vi "SwitchToAnalogOrDigital.vi"(0 "System no.":i32=1 min=1 step=1, 1 "Controller analog board":enum16{"E-711.iA4"}(ring), 2 "Axes to command":string[](array[string]), 3 "Mode":bool=TRUE caption="Mode (Analog:T)", 5 "error in":errorcluster, 6 "AI channels":dbl[](array[numeric]), 7 "AO channels":dbl[](array[numeric]), 8 "Lower voltage limit (V)":dbl=-10.0 format="%.6f", 9 "Upper voltage limit (V)":dbl=10.0 format="%.6f") -> (14 "Conversion factor":dbl[](array[numeric]) format="%.2f", 15 "Offset":dbl[](array[numeric]) format="%#.6f", 19 "Error out":errorcluster)   [LabVIEW 2014, in "PiFOC.lvlib"]
doc: "This VI sets communication parameters for analog or digital control. Run XXXX_Configuration_Setup.vi (with XXXX being the product number of your PI controller) prior to running this VI. \n\n¢ Set System no. to the same value as selected in XXXX_Configuration_ Setup.vi. \n¢ Select the name of the controller analog board (E-711.iA4).\n¢ Mode can be Analog (T) or Digital (F). \n¢ Lower voltage limit (V) and Upper voltage limit (V) must match the corresponding settings in Analog_Configuration_Setup.vi, representing the voltage range of the analog input of the controller. The VI checks if the selected values fit into the analog input voltage range of the controller. \n¢ Axes to command must be a sub set of the axes connected to the controller. \n¢ AI channels are the analog input channels of the controller to use for analog control. In contrast to the firmware internal names of the analog input channels, select \"1\" here for the first analog input, \"2\" for the second and so on. The VI will automatically determine which input channel names correspond to the selected analog input channels. \n¢ Similarly, select \"1\" for the first analog output channel (AO channels), \"2\" for the second analog output channel and so on, as the VI will automatically determine which output channel names correspond to the selected analog output channels. \n\nIf the current command level is 0 (CCL?), the VI switches to command level 1 (CCL) before making any further settings and back to 0 afterwards. \nWhen Analog is selected as Mode, the VI connects the selected analog input channels to the selected axes (SPA), sets gain and offset for the analog input (SPA), sets the output type to sensor monitor output (SPA), connects the selected analog output channels to the selected axes (SPA), and sets the position report scaling value and offset for the analog output (SPA).\nWhen Digital is selected as Mode, the VI disconnects the selected analog input channels from the axes (SPA) and sets the output type to control output (SPA).\nThe VI returns the total number of input and output channels available for this controller, the number of sensor input/output channels and the resulting number of analog input/output channels available for analog control. Also, it returns the Gain, Offset and Conversion factor settings resulting from the motion range (TMX?, TMN?) of the selected axes and sets the corresponding parameters (SPA). Finally, it returns the minimum and maximum analog input voltages of the controller as the given lower and upper voltage limits must fit into this range.\n\nSee XXXX_Sample_Application_With_Analog.vi (with XXXX being the product number of your PI controller) as a sample VI showing how to use this VI in combination with the corresponding Configuration_Setup VIs. \n\nValid for: E-709, E-712, E-725\n\nE-709: Controller analog board selection is E-711.iA4 (but board has different product code). \nE-712: Controller analog board is E-711.iA\nE-725: Controller analog board selection is E-711.iA4 (but board has different product code)."
uses:
  PiFOC.lvlib
panel:
  out "Max. controller\nanalog input voltage":dbl format="%#.6f"
  out "Min. controller\nanalog input voltage":dbl format="%#.6f"
  out "Gain":dbl[](array[numeric]) format="%#.6f"
  out "No. of output channels":dbl format="%#.0f"
  out "No. of sensor output channels":dbl format="%#.0f"
  out "No. of AO channels":dbl format="%#.0f"
  out "No. of AI channels":dbl format="%#.0f"
  out "No. of sensor input channels":dbl format="%#.0f"
  out "No. of input channels":dbl format="%#.0f"
  # "This VI sets communication parameters for analog or digital control. Run XXXX_Configuration_Setup.vi (with XXXX being the \nproduct number of your PI controller) prior to running this VI. Set System no. to the same value as selected in XXXX_Configu-\nration_Setup.vi. See online help for details."
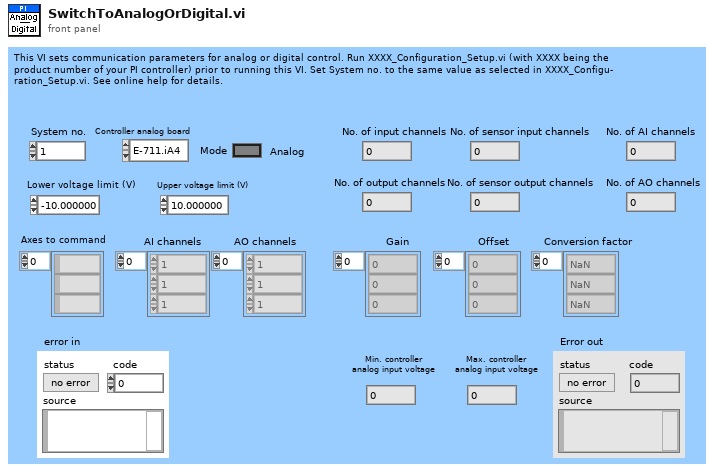
[diagram p1: front panel]
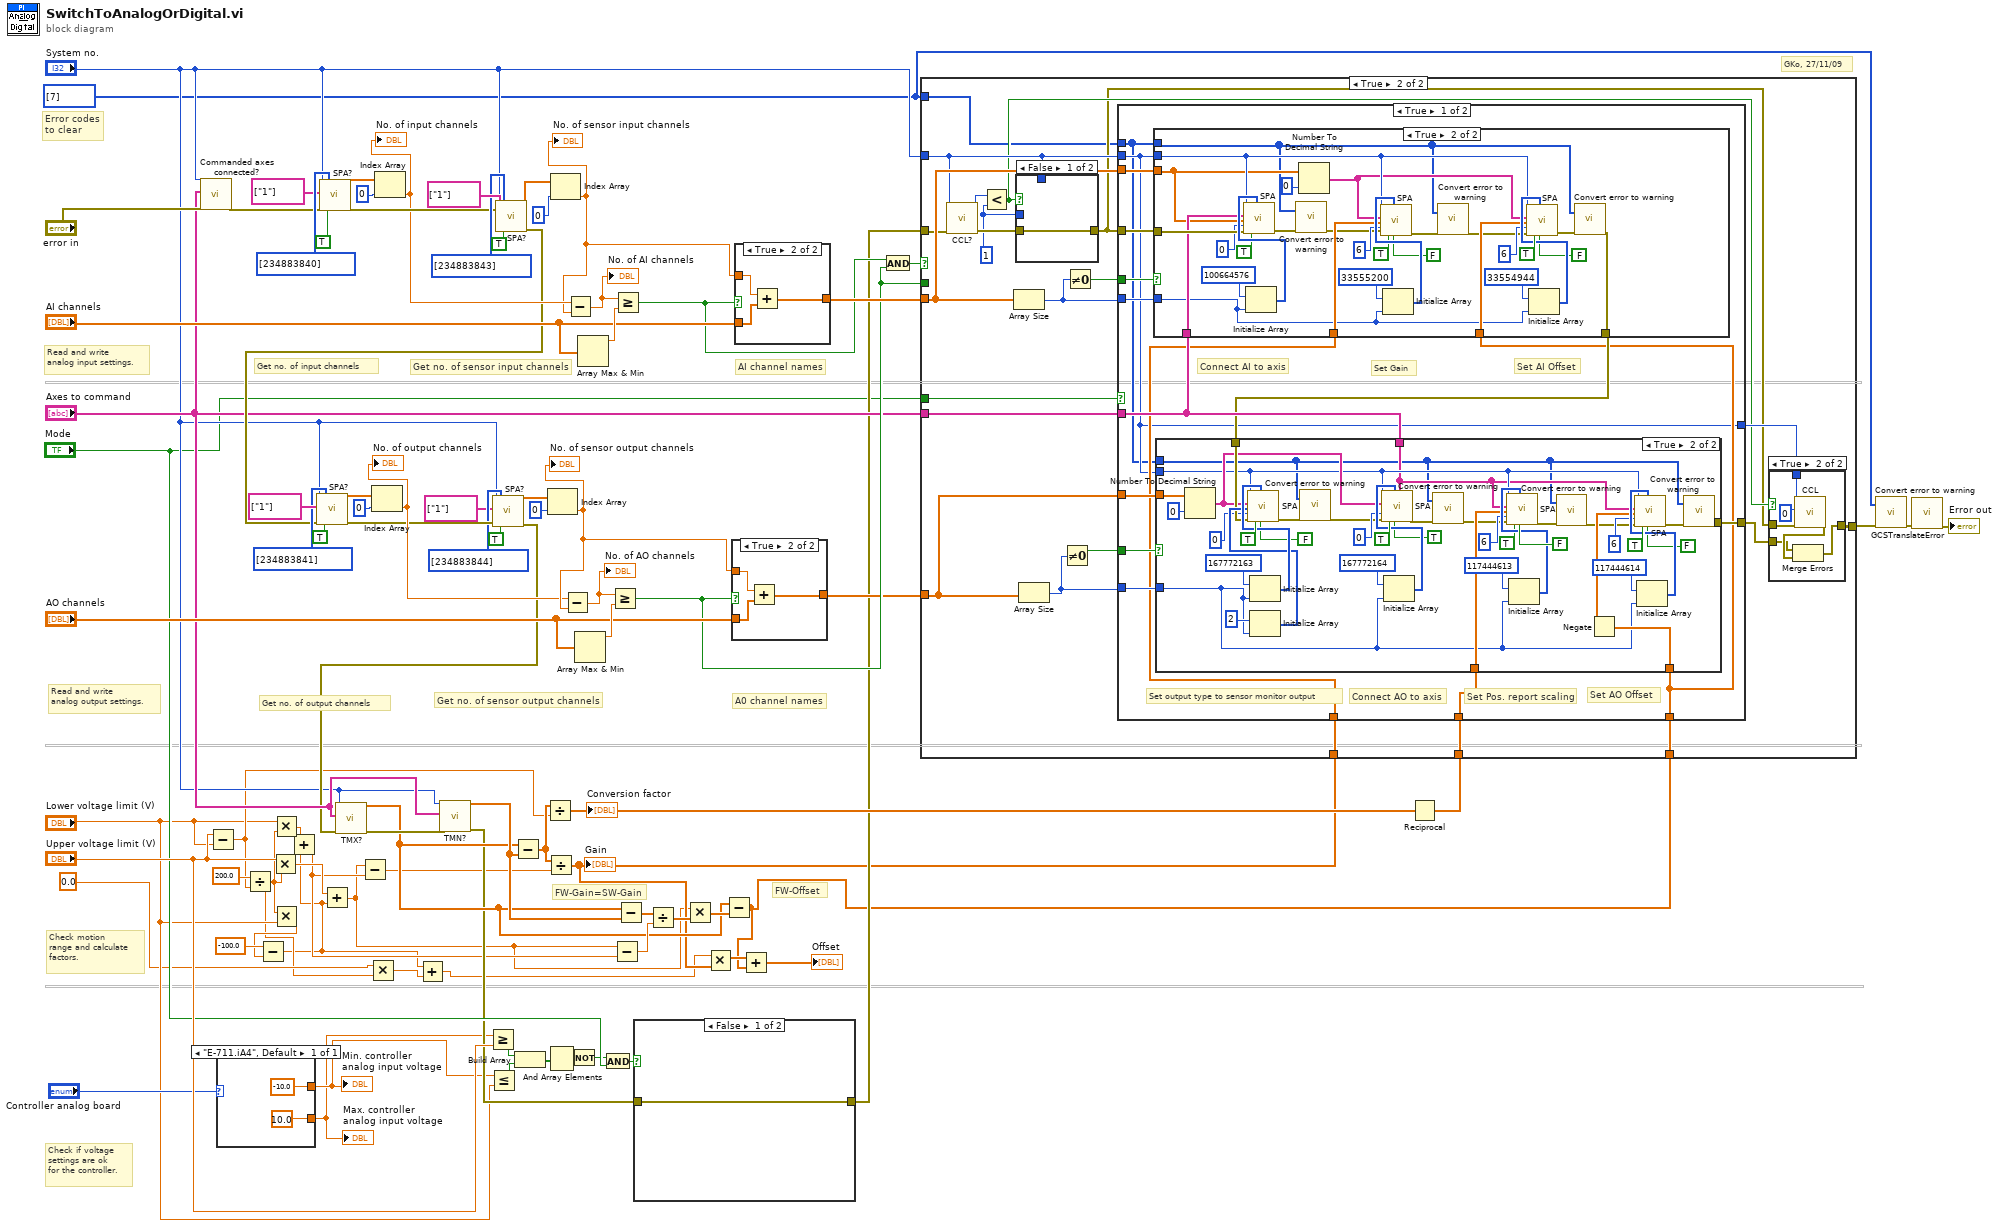
[diagram p0: block diagram]
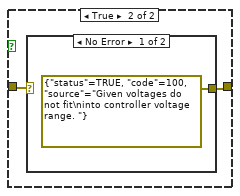
[diagram p2: hidden frame]
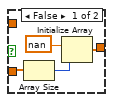
[diagram p4: hidden frame]
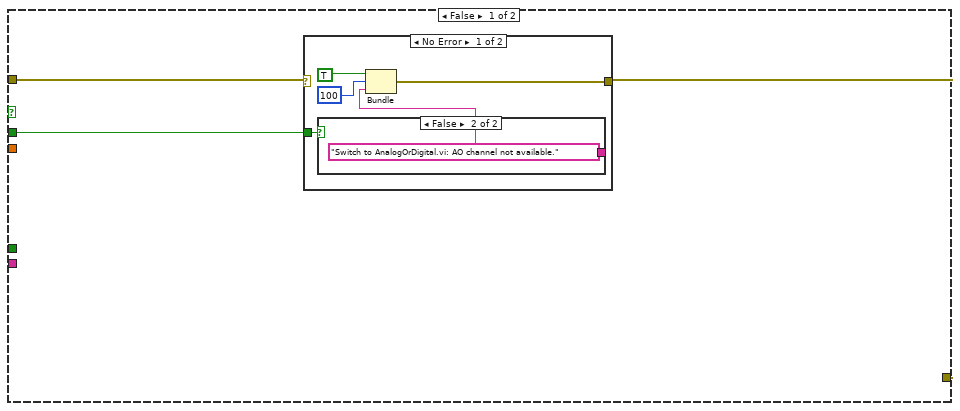
[diagram p5: hidden frame]
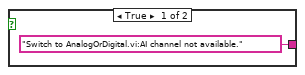
[diagram p6: hidden frame]
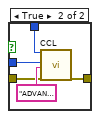
[diagram p9: hidden frame]
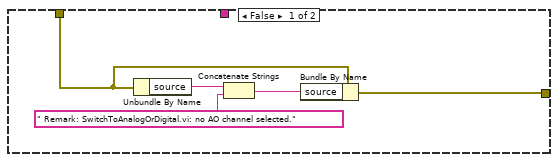
[diagram p10: hidden frame]
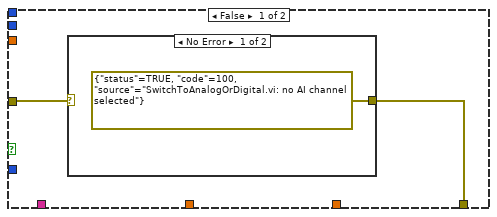
[diagram p11: hidden frame]
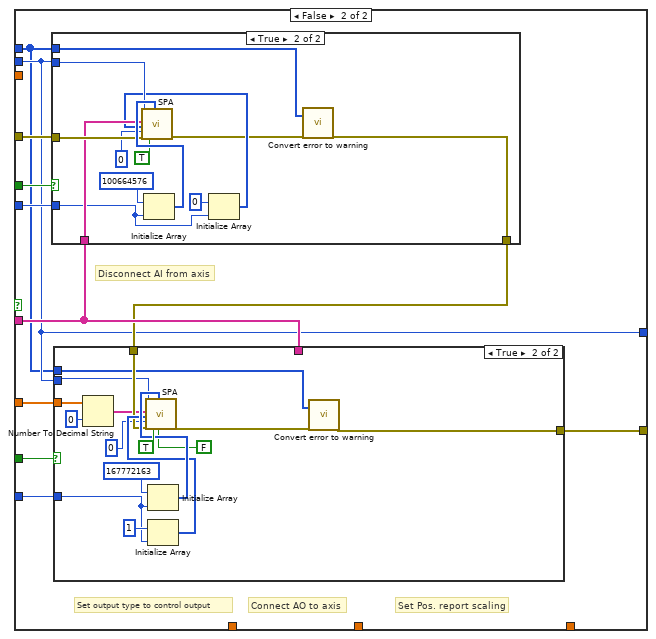
[diagram p13: hidden frame]
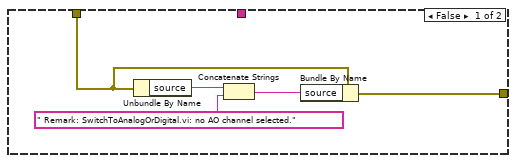
[diagram p14: hidden frame]
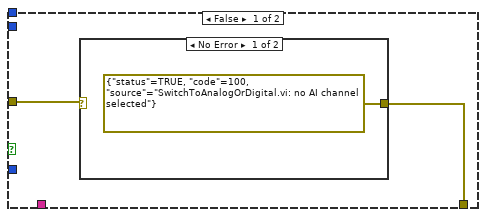
[diagram p15: hidden frame]
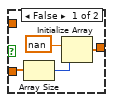
[diagram p17: hidden frame]
diagram:
  w20 = i32[] [7] ("Codes")
  # "Error codes\nto clear"
  # "Get no. of sensor output channels"
  # "Get no. of output channels"
  # "Get no. of sensor input channels"
  # "Get no. of input channels"
  # "FW-Offset"
  # "FW-Gain=SW-Gain"
  # "A0 channel names"
  # "GKo, 27/11/09"
  # "Read and write\nanalog output settings."
  # "Check motion\nrange and calculate\nfactors."
  # "Check if voltage\nsettings are ok\nfor the controller."
  # "AI channel names"
  # "Read and write\nanalog input settings."
  n1 = call "Commanded axes connected?.vi"("System no."="System no.", "Commanded axes"="Axes to command", "error in"="error in") -> ("error out"=w73:errorcluster)  [unwired: 16 out]
  n2 = Subtract(x="Upper voltage limit (V)", y="Lower voltage limit (V)") -> (x-y=w18:dbl)
  n3 = case shown="\"E-711.iA4\", Default" "Controller analog board" {
    tunnel: [-10.0 ("y")] -> w25
    tunnel: [10.0 ("y")] -> w24
    frame "E-711.iA4", Default {
    }
  }
  "Min. controller\nanalog input voltage" <- w25
  "Max. controller\nanalog input voltage" <- w24
  n4 = Divide(x=200.0, y=w18) -> (x/y=w3:dbl)
  n5 = Multiply(x="Upper voltage limit (V)", y=w3) -> (x*y=w13:dbl)
  n6 = Multiply(x="Lower voltage limit (V)", y=w3) -> (x*y=w14:dbl)
  n7 = Multiply(x=w3, y="Lower voltage limit (V)") -> (x*y=w15:dbl)
  n8 = Subtract(x=-100.0, y=w15) -> (x-y=w2:dbl)
  n9 = Add(x=w14, y=w2) -> (x+y=w7:dbl)
  n10 = call "SPA?.vi"("System no."="System no.", "Axes to query"=string[] ["1"], "error in"=w73, "Parameter no. (hex)"=u32[] [234883840], "Parameter no. format \n(Decimal: FALSE)"=TRUE ("Parameter no. format \n(Decimal: FALSE)")) -> ("Parameter value"=w86:dbl[], "error out"=w79:errorcluster)  [unwired: 2 in, 11 out]
  n11 = Add(x=w13, y=w2) -> (x+y=w6:dbl)
  n12 = Subtract(x=w6, y=w7) -> (x-y=w4:dbl)
  n13 = Multiply(x=0.0, y=w3) -> (x*y=w5:dbl)
  n14 = Index Array(array=w86, index=0) -> (element=w78:dbl)
  "No. of input channels" <- w78
  n15 = Add(x=w2, y=w5) -> (x+y=w1:dbl)
  n16 = Greater Or Equal?(x=w24, y="Upper voltage limit (V)") -> (x >= y?=w35:bool)
  n17 = Less Or Equal?(x=w25, y="Lower voltage limit (V)") -> (x <= y?=w34:bool)
  n18 = call "SPA?.vi"("System no."="System no.", "Axes to query"=string[] ["1"], "error in"=w79, "Parameter no. (hex)"=u32[] [234883843], "Parameter no. format \n(Decimal: FALSE)"=TRUE ("Parameter no. format \n(Decimal: FALSE)")) -> ("Parameter value"=w83:dbl[], "error out"=w55:errorcluster)  [unwired: 2 in, 11 out]
  n19 = call "SPA?.vi"("System no."="System no.", "Axes to query"=string[] ["1"], "error in"=w55, "Parameter no. (hex)"=u32[] [234883841], "Parameter no. format \n(Decimal: FALSE)"=TRUE ("Parameter no. format \n(Decimal: FALSE)")) -> ("Parameter value"=w59:dbl[], "error out"=w66:errorcluster)  [unwired: 2 in, 11 out]
  n20 = Index Array(array=w59, index=0) -> (element=w67:dbl)
  "No. of output channels" <- w67
  n21 = call "SPA?.vi"("System no."="System no.", "Axes to query"=string[] ["1"], "error in"=w66, "Parameter no. (hex)"=u32[] [234883844], "Parameter no. format \n(Decimal: FALSE)"=TRUE ("Parameter no. format \n(Decimal: FALSE)")) -> ("Parameter value"=w62:dbl[], "error out"=w49:errorcluster)  [unwired: 2 in, 11 out]
  n22 = call "TMX?.vi"("System no."="System no.", "Axes to query"="Axes to command", "error in"=w49) -> ("Maximum travel limit"=w42:dbl[], "error out"=w48:errorcluster)  [unwired: 2 in, 13 out]
  n23 = call "TMN?.vi"("System no."="System no.", "Axes to query"="Axes to command", "error in"=w48) -> ("Minimum travel limit"=w47:dbl[], "error out"=w26:errorcluster)  [unwired: 2 in, 13 out]
  n24 = Subtract(x=w42, y=w47) -> (x-y=w41:dbl[])
  n25 = Build Array(w35, w34) -> (w33:bool[])
  n26 = Divide(x=w41, y=w18) -> (x/y=w40:dbl[])
  "Conversion factor" <- w40
  n27 = Divide(x=w41, y=w4) -> (x/y=w12:dbl[])
  "Gain" <- w12
  n28 = And Array Elements(Boolean array=w33) -> (logical AND=w30:bool)
  n29 = Index Array(array=w62, index=0) -> (element=w68:dbl)
  "No. of sensor output channels" <- w68
  n30 = Index Array(array=w83, index=0) -> (element=w77:dbl)
  "No. of sensor input channels" <- w77
  n31 = Subtract(x=w67, y=w68) -> (x-y=w69:dbl)
  "No. of AO channels" <- w69
  n32 = Subtract(x=w78, y=w77) -> (x-y=w76:dbl)
  "No. of AI channels" <- w76
  n33 = Not(x=w30) -> (.not. x?=w28:bool)
  n34 = Array Max & Min(array="AO channels") -> (max value=w70:dbl)  [unwired: 3 out]
  n35 = Array Max & Min(array="AI channels") -> (max value=w75:dbl)  [unwired: 3 out]
  n36 = And(x=w28, y="Mode") -> (x .and. y?=w27:bool)
  n37 = Greater Or Equal?(x=w69, y=w70) -> (x >= y?=w51:bool)
  n38 = Subtract(x=w6, y=w7) -> (x-y=w45:dbl)
  n39 = Greater Or Equal?(x=w76, y=w75) -> (x >= y?=w53:bool)
  n40 = Subtract(x=w42, y=w47) -> (x-y=w46:dbl[])
  n41 = case shown="False" w27 {
    tunnel: w26 -> [w92 w94]
    tunnel: [w92 w93] -> w32
    frame False {
    }
    frame True {
      n42 = case shown="No Error" w94 {
        selector: w94 -> [_ w96]
        tunnel: [errorcluster {"status"=TRUE, "code"=100, "source"="Given voltages do not fit\ninto controller voltage range. "} ("error IO") w96] -> w93
        frame No Error {
        }
        frame Error {
        }
      }
    }
  }
  n43 = Divide(x=w46, y=w45) -> (x/y=w44:dbl[])
  n44 = Multiply(x=w6, y=w44) -> (x*y=w43:dbl[])
  n45 = Multiply(x=w1, y=w12) -> (x*y=w11:dbl[])
  n46 = Subtract(x=w42, y=w43) -> (x-y=w10:dbl[])
  n47 = case shown="True" w51 {
    tunnel: "AO channels" -> [w100 w102]
    tunnel: w68 -> [_ w103]
    tunnel: [w97 w101] -> w38
    frame False {
      n48 = Array Size(array=w100) -> (size(s)=w98:i32)
      n49 = Initialize Array(nan, w98) -> (w97:dbl[])
    }
    frame True {
      n50 = Add(x=w103, y=w102) -> (x+y=w101:dbl[])
    }
  }
  n51 = case shown="True" w53 {
    tunnel: "AI channels" -> [w107 w109]
    tunnel: w77 -> [_ w110]
    tunnel: [w104 w108] -> w71
    frame False {
      n52 = Array Size(array=w107) -> (size(s)=w105:i32)
      n53 = Initialize Array(nan, w105) -> (w104:dbl[])
    }
    frame True {
      n54 = Add(x=w110, y=w109) -> (x+y=w108:dbl[])
    }
  }
  n55 = Add(x=w11, y=w10) -> (x+y=→"Offset":dbl[])
  n56 = And(x=w53, y=w51) -> (x .and. y?=w52:bool)
  n57 = Reciprocal(x=w40) -> (1/x=w39:dbl[])
  n58 = case shown="True" w52 {
    tunnel: "System no." -> [_ w128]
    tunnel: w71 -> [_ w133]
    tunnel: "Axes to command" -> [_ w142]
    tunnel: w32 -> [w113 w129]
    tunnel: w51 -> [w112 _]
    tunnel: w38 -> [_ w143]
    tunnel: w12 -> [_ w136]
    tunnel: w10 -> [_ w135]
    tunnel: [w111 w132] -> w22
    tunnel: w39 -> [_ w141]
    tunnel: "Mode" -> [_ w134]
    tunnel: w20 -> [_ w122]
    frame False {
      n59 = case shown="No Error" w113 {
        selector: w113 -> [_ w121]
        tunnel: w112 -> [w116 _]
        tunnel: [w114 w121] -> w111
        frame No Error {
          n60 = case shown="False" w116 {
            tunnel: ["Switch to AnalogOrDigital.vi:AI channel not available." ("source") "Switch to AnalogOrDigital.vi: AO channel not available." ("source")] -> w115
            frame True {
            }
            frame False {
            }
          }
          n61 = Bundle("status"=TRUE, "code"=100, "source"=w115) -> (w114:errorcluster)  [unwired: 1 out]
        }
        frame Error {
        }
      }
    }
    frame True {
      w126 = 1 ("Command level")
      n62 = call "CCL?.vi"("System no."=w128, "error in"=w129) -> ("Command level"=w127:i32, "error out"=w130:errorcluster)  [unwired: 16 out]
      n63 = Less?(x=w127, y=w126) -> (x < y?=w125:bool)
      n64 = Array Size(array=w133) -> (size(s)=w139:i32)
      n65 = case shown="False" w125 {
        tunnel: [w151 w156] -> w124
        tunnel: w130 -> [w151 w154]
        tunnel: w128 -> [_ w153]
        tunnel: w126 -> [_ w152]
        frame False {
        }
        frame True {
          n66 = call "CCL.vi"("System no."=w153, "Command level"=w152, "Password"="ADVANCED", "error in"=w154) -> ("error out"=w156:errorcluster)  [unwired: 15 out]
        }
      }
      n67 = Array Size(array=w143) -> (size(s)=w138:i32)
      n68 = Not Equal To 0?(x=w138) -> (x != 0?=w137:bool)
      n69 = Not Equal To 0?(x=w139) -> (x != 0?=w140:bool)
      n70 = case shown="True" w134 {
        tunnel: w124 -> [w171 w262]
        tunnel: w143 -> [w170 w261]
        tunnel: [w169 w260] -> w123
        tunnel: w142 -> [w168 w259]
        tunnel: w141 -> [w167 _]
        tunnel: w128 -> [w158 w253]
        tunnel: w133 -> [w165 _]
        tunnel: w140 -> [w164 w257]
        tunnel: w139 -> [w163 w256]
        tunnel: w138 -> [w162 w255]
        tunnel: w137 -> [w161 w254]
        tunnel: w136 -> [w160 _]
        tunnel: w135 -> [w159 _]
        tunnel: [w158 w253] -> w131
        tunnel: w122 -> [w157 w252]
        frame True {
          # "Set AO Offset"
          # "Set Pos. report scaling"
          # "Set AI Offset"
          # "Set Gain"
          # "Connect AO to axis"
          # "Set output type to sensor monitor output"
          # "Connect AI to axis"
          n71 = case shown="True" w164 {
            tunnel: w171 -> [w219 w249]
            tunnel: w160 -> [_ w244]
            tunnel: w159 -> [_ w238]
            tunnel: w168 -> [_ w237]
            tunnel: [w218 w223] -> w166
            tunnel: w158 -> [_ w236]
            tunnel: w163 -> [_ w235]
            tunnel: w165 -> [_ w233]
            tunnel: w157 -> [_ w222]
            frame False {
              n72 = case shown="No Error" w219 {
                selector: w219 -> [_ w221]
                tunnel: [errorcluster {"status"=TRUE, "code"=100, "source"="SwitchToAnalogOrDigital.vi: no AI channel selected"} ("error IO") w221] -> w218
                frame No Error {
                }
                frame Error {
                }
              }
            }
            frame True {
              n73 = Initialize Array(100664576 ("Numeric"), w235) -> (w250:i32[])
              n74 = call "SPA.vi"("System no."=w236, "Axis to set"=w237, "Parameter value"=w233, "No.of digits"=i16 0, "error in"=w249, "Parameter no. format \n(Decimal: FALSE)"=TRUE ("Parameter no. format \n(Decimal: FALSE)"), "Parameter number (hex)"=w250) -> ("error out"=w228:errorcluster)  [unwired: 3 in, 9 out]
              n75 = call "Convert error to warning.vi"("Codes"=w222, "error in"=w228) -> ("error out"=w227:errorcluster)  [unwired: 17 out]
              n76 = Number To Decimal String(number=w233, width (-)=i16 0) -> (decimal integer string=w234:string[])
              n77 = Initialize Array(33555200 ("Numeric"), w235) -> (w246:i32[])
              n78 = call "SPA.vi"("System no."=w236, "Axis to set"=w234, "Parameter value"=w244, "No.of digits"=i16 6, "error in"=w227, "Parameter no. format \n(Decimal: FALSE)"=TRUE ("Parameter no. format \n(Decimal: FALSE)"), "Parameter number (hex)"=w246, "Parameter format \n(Num.: FALSE)"=FALSE ("Parameter format \n(Num.: FALSE)")) -> ("error out"=w226:errorcluster)  [unwired: 2 in, 9 out]
              n79 = call "Convert error to warning.vi"("Codes"=w222, "error in"=w226) -> ("error out"=w225:errorcluster)  [unwired: 17 out]
              n80 = Initialize Array(33554944 ("Numeric"), w235) -> (w242:i32[])
              n81 = call "SPA.vi"("System no."=w236, "Axis to set"=w234, "Parameter value"=w238, "No.of digits"=i16 6, "error in"=w225, "Parameter no. format \n(Decimal: FALSE)"=TRUE ("Parameter no. format \n(Decimal: FALSE)"), "Parameter number (hex)"=w242, "Parameter format \n(Num.: FALSE)"=FALSE ("Parameter format \n(Num.: FALSE)")) -> ("error out"=w224:errorcluster)  [unwired: 2 in, 9 out]
              n82 = call "Convert error to warning.vi"("Codes"=w222, "error in"=w224) -> ("error out"=w223:errorcluster)  [unwired: 17 out]
            }
          }
          n83 = case shown="True" w161 {
            tunnel: w170 -> [_ w209]
            tunnel: [w172 w178] -> w169
            tunnel: w168 -> [_ w191]
            tunnel: w167 -> [_ w202]
            tunnel: w166 -> [w173 w201]
            tunnel: w158 -> [_ w194]
            tunnel: w162 -> [_ w186]
            tunnel: w159 -> [_ w193]
            tunnel: w157 -> [_ w177]
            frame False {
              n84 = Unbundle By Name(w173) -> ("source"=w176:string)
              n85 = Concatenate Strings(w176, " Remark: SwitchToAnalogOrDigital.vi: no AO channel selected." ("source")) -> (w174:string)
              n86 = Bundle By Name(cluster=w173, "source"=w174) -> (w172:errorcluster)
            }
            frame True {
              n87 = Number To Decimal String(number=w209, width (-)=i16 0) -> (decimal integer string=w200:string[])
              n88 = Initialize Array(167772163 ("Numeric"), w186) -> (w216:i32[])
              n89 = Initialize Array(2 ("element"), w186) -> (w213:i32[])
              n90 = call "SPA.vi"("System no."=w194, "Axis to set"=w200, "Parameter value"=w213, "No.of digits"=i16 0, "error in"=w201, "Parameter no. format \n(Decimal: FALSE)"=TRUE ("Parameter no. format \n(Decimal: FALSE)"), "Parameter number (hex)"=w216, "Parameter format \n(Num.: FALSE)"=FALSE ("Parameter format \n(Num.: FALSE)")) -> ("error out"=w185:errorcluster)  [unwired: 2 in, 9 out]
              n91 = call "Convert error to warning.vi"("Codes"=w177, "error in"=w185) -> ("error out"=w184:errorcluster)  [unwired: 17 out]
              n92 = Initialize Array(167772164 ("Numeric"), w186) -> (w211:i32[])
              n93 = call "SPA.vi"("System no."=w194, "Axis to set"=w200, "No.of digits"=i16 0, "error in"=w184, "Parameter no. format \n(Decimal: FALSE)"=TRUE ("Parameter no. format \n(Decimal: FALSE)"), "Parameter number (hex)"=w211, "Parameter format \n(Num.: FALSE)"=TRUE ("Parameter format \n(Num.: FALSE)"), "Parameter string"=w191) -> ("error out"=w183:errorcluster)  [unwired: 2 in, 9 out]
              n94 = call "Convert error to warning.vi"("Codes"=w177, "error in"=w183) -> ("error out"=w182:errorcluster)  [unwired: 17 out]
              n95 = Initialize Array(117444613 ("Numeric"), w186) -> (w204:i32[])
              n96 = call "SPA.vi"("System no."=w194, "Axis to set"=w191, "Parameter value"=w202, "No.of digits"=i16 6, "error in"=w182, "Parameter no. format \n(Decimal: FALSE)"=TRUE ("Parameter no. format \n(Decimal: FALSE)"), "Parameter number (hex)"=w204, "Parameter format \n(Num.: FALSE)"=FALSE ("Parameter format \n(Num.: FALSE)")) -> ("error out"=w180:errorcluster)  [unwired: 2 in, 9 out]
              n97 = call "Convert error to warning.vi"("Codes"=w177, "error in"=w180) -> ("error out"=w181:errorcluster)  [unwired: 17 out]
              n98 = Negate(x=w193) -> (-x=w192:dbl[])
              n99 = Initialize Array(117444614 ("Numeric"), w186) -> (w197:i32[])
              n100 = call "SPA.vi"("System no."=w194, "Axis to set"=w191, "Parameter value"=w192, "No.of digits"=i16 6, "error in"=w181, "Parameter no. format \n(Decimal: FALSE)"=TRUE ("Parameter no. format \n(Decimal: FALSE)"), "Parameter number (hex)"=w197, "Parameter format \n(Num.: FALSE)"=FALSE ("Parameter format \n(Num.: FALSE)")) -> ("error out"=w179:errorcluster)  [unwired: 2 in, 9 out]
              n101 = call "Convert error to warning.vi"("Codes"=w177, "error in"=w179) -> ("error out"=w178:errorcluster)  [unwired: 17 out]
            }
          }
        }
        frame False {
          # "Set Pos. report scaling"
          # "Connect AO to axis"
          # "Set output type to control output"
          # "Disconnect AI from axis"
          n102 = case shown="True" w257 {
            tunnel: w262 -> [w285 w298]
            tunnel: w259 -> [_ w296]
            tunnel: [w284 w290] -> w258
            tunnel: w253 -> [_ w295]
            tunnel: w256 -> [_ w294]
            tunnel: w252 -> [_ w288]
            frame False {
              n103 = case shown="No Error" w285 {
                selector: w285 -> [_ w287]
                tunnel: [errorcluster {"status"=TRUE, "code"=100, "source"="SwitchToAnalogOrDigital.vi: no AI channel selected"} ("error IO") w287] -> w284
                frame No Error {
                }
                frame Error {
                }
              }
            }
            frame True {
              n104 = Initialize Array(100664576 ("Numeric"), w294) -> (w299:i32[])
              n105 = Initialize Array(0 ("element"), w294) -> (w292:i32[])
              n106 = call "SPA.vi"("System no."=w295, "Axis to set"=w296, "Parameter value"=w292, "No.of digits"=i16 0, "error in"=w298, "Parameter no. format \n(Decimal: FALSE)"=TRUE ("Parameter no. format \n(Decimal: FALSE)"), "Parameter number (hex)"=w299) -> ("error out"=w289:errorcluster)  [unwired: 3 in, 9 out]
              n107 = call "Convert error to warning.vi"("Codes"=w288, "error in"=w289) -> ("error out"=w290:errorcluster)  [unwired: 17 out]
            }
          }
          n108 = case shown="True" w254 {
            tunnel: w261 -> [_ w278]
            tunnel: [w263 w270] -> w260
            tunnel: w259 -> [_ _]
            tunnel: w258 -> [w267 w276]
            tunnel: w253 -> [_ w275]
            tunnel: w255 -> [_ w274]
            tunnel: w252 -> [_ w268]
            frame False {
              n109 = Unbundle By Name(w267) -> ("source"=w266:string)
              n110 = Concatenate Strings(w266, " Remark: SwitchToAnalogOrDigital.vi: no AO channel selected." ("source")) -> (w264:string)
              n111 = Bundle By Name(cluster=w267, "source"=w264) -> (w263:errorcluster)
            }
            frame True {
              n112 = Number To Decimal String(number=w278, width (-)=i16 0) -> (decimal integer string=w273:string[])
              n113 = Initialize Array(167772163 ("Numeric"), w274) -> (w282:i32[])
              n114 = Initialize Array(1 ("element"), w274) -> (w279:i32[])
              n115 = call "SPA.vi"("System no."=w275, "Axis to set"=w273, "Parameter value"=w279, "No.of digits"=i16 0, "error in"=w276, "Parameter no. format \n(Decimal: FALSE)"=TRUE ("Parameter no. format \n(Decimal: FALSE)"), "Parameter number (hex)"=w282, "Parameter format \n(Num.: FALSE)"=FALSE ("Parameter format \n(Num.: FALSE)")) -> ("error out"=w269:errorcluster)  [unwired: 2 in, 9 out]
              n116 = call "Convert error to warning.vi"("Codes"=w268, "error in"=w269) -> ("error out"=w270:errorcluster)  [unwired: 17 out]
            }
          }
        }
      }
      n117 = case shown="True" w125 {
        tunnel: [w144 w145] -> w132
        tunnel: w131 -> [_ w150]
        tunnel: w124 -> [_ w148]
        tunnel: w123 -> [w144 w146]
        frame False {
        }
        frame True {
          n118 = call "CCL.vi"("System no."=w150, "Command level"=0, "error in"=w148) -> ("error out"=w147:errorcluster)  [unwired: 1 in, 15 out]
          n119 = Merge Errors(w146, w147) -> (w145:errorcluster)
        }
      }
    }
  }
  n120 = call "Convert error to warning.vi"("Codes"=w20, "error in"=w22) -> ("error out"=w21:errorcluster)  [unwired: 17 out]
  n121 = call "GCSTranslateError.vi"("error in"=w21) -> ("error out"=→"Error out":errorcluster)  [unwired: 18 out]
